vi "Insert SubPanel.vi"(8 "error in (no error)":errorcluster, 9 "ActorQName":string, 10 "ActorVI Ref":refnum<vi>, 11 "CheckPasswordUI in":refnum<class "CheckPasswordUI.lvclass">) -> (0 "error out":errorcluster, 3 "CheckPasswordUI out":refnum<class "CheckPasswordUI.lvclass">)   [LabVIEW 2021, in "CheckPasswordUI.lvclass"]
uses:
  CheckPasswordUI.lvclass
  C:/Program Files (x86)/National Instruments/LabVIEW 2021/vi.lib/ActorFramework/Actor/Actor.lvclass
  <vilib>/ActorFramework/Actor/Actor.lvclass/Actor.ctl
  <userlib>/John_Lib/Interfaces/InsertRightSubPanel Messages/Insert Right SubPanel Msg/Insert Right SubPanel Msg.lvclass/Insert Right SubPanel Msg.ctl
  <vilib>/ActorFramework/Message Enqueuer/Message Enqueuer.lvclass/Message Enqueuer.ctl
  <vilib>/ActorFramework/Message Enqueuer/Enqueue.vi
  <userlib>/John_Lib/Interfaces/InsertRightSubPanel Messages/Insert Right SubPanel Msg/Insert Right SubPanel Msg.lvclass
  C:/Program Files (x86)/National Instruments/LabVIEW 2021/vi.lib/ActorFramework/Message/Message.lvclass
  <vilib>/ActorFramework/Message Priority Queue/Priority Enqueue.vi
  <vilib>/ActorFramework/Actor/Actor.lvclass
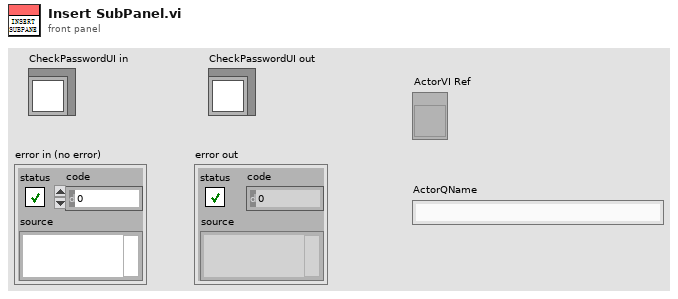
[diagram p1: front panel]
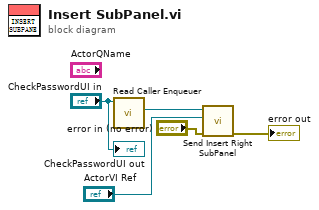
[diagram p0: block diagram]
diagram:
  n1 = call <vilib>:"Read Caller Enqueuer.vi"("Actor"="CheckPasswordUI in") -> ("Caller Enqueuer"=w4:refnum<class "Message Enqueuer.lvclass">)  [unwired: 10 in]
  n2 = call <userlib>:"Send Insert Right SubPanel.vi"("error in (no error)"="error in (no error)", "ActorVI Ref"="ActorVI Ref", "Message Enqueuer"=w4) -> ("error out"=→"error out":errorcluster)  [unwired: 7 in, 1 out]
  "CheckPasswordUI out" <- "CheckPasswordUI in"
